vi "Teleop.vi"(10 "Match Info":T1={"Autonomous Elapsed Seconds"=0.0, "TeleOp Elapsed Seconds"=0.0, "Disabled Elapsed Seconds"=0.0, "Visited Autonomous"=FALSE, "Visited TeleOp"=FALSE, "Visited Disabled"=FALSE, "Autonomous Settings"={"Autonomous Style"=enum."Independent", "VI Refnum"=refnum}}, 11 "Call Context":T2) -> ()   [LabVIEW 2011]
doc: "This VI is called for each TeleOp packet received from the DS where the robot is not disabled. It is often used to read from the joysticks and update I/O or to update setpoints for timed control loops. It should complete and return within 20 milliseconds or it may miss DS packets."
uses:
  <vilib>/Rock Robotics/WPI/DriverStation/WPI_DriverStationDerivedRobotMode.ctl
  <vilib>/Rock Robotics/WPI/DriverStation/WPI_DriverStationMatch Info.ctl
  Robot Global Data.vi
panel:
  out "Right Speed":dbl
  out "Left Speed":dbl
  out "Hammer Speed":dbl
  out "Angle Speed":dbl
  in  "Test Shooter":bool
  out "Collector Speed":dbl
  out "Elevator Speed":dbl
  out "Shooter Speed":dbl
  # "Motot Inputs"
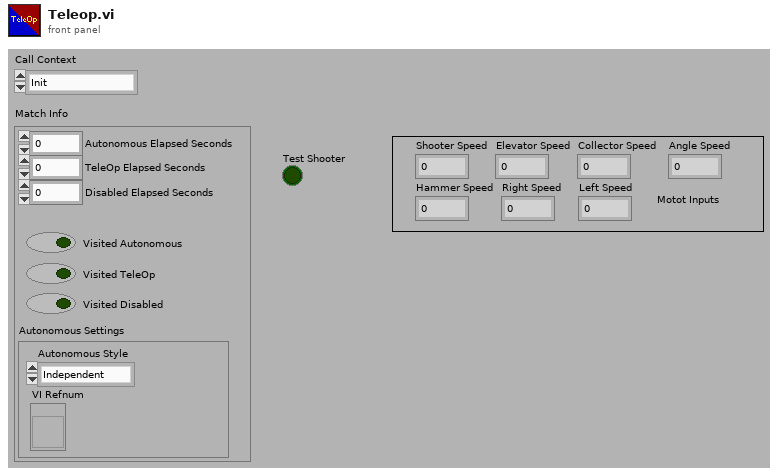
[diagram p1: front panel]
types:
  T1 = typedef "WPI_DriverStationMatch Info.ctl" = cluster{"Autonomous Elapsed Seconds":dbl, "TeleOp Elapsed Seconds":dbl, "Disabled Elapsed Seconds":dbl, "Visited Autonomous":bool, "Visited TeleOp":bool, "Visited Disabled":bool, "Autonomous Settings":cluster{"Autonomous Style":enum16{"Iterative", "Independent"}, "VI Refnum":refnum<vi>}}
  T2 = typedef "WPI_DriverStationDerivedRobotMode.ctl" = enum16{"Init", "Execute", "Stop"}
  T3 = typedef "WPI_JoystickDevRef.ctl" = cluster{"Device":T4}
  T4 = typedef "WPI_JoystickDeviceEnum.ctl" = enum16{"USB 1", "USB 2", "USB 3", "USB 4", "Kinect 1", "Kinect 2"}
  T5 = typedef "WPI_JoystickButtonState.ctl" = cluster{"Button 1":bool, "Button 2":bool, "Button 3":bool, "Button 4":bool, "Button 5":bool, "Button 6":bool, "Button 7":bool, "Button 8":bool, "Button 9":bool, "Button 10":bool, "Button 11":bool, "Button 12":bool}
  T6 = cluster{"axis 1 (x)":dbl, "axis 2 (y)":dbl, "axis 3 (throttle)":dbl, "axis 4":dbl, "axis 5":dbl, "axis 6":dbl}
  T7 = typedef "WPI_MotorControlDeviceRef.ctl" = cluster{"DeviceStatus":errorcluster, "Type":enum16{"PWM", "CAN"}, "PWM":cluster{"Digital Module":T8, "PWM Channel":T9, "DeadBand":T10}, "CAN":cluster{"Device Number":u8, "Control Mode":T11, "Semaphore":T12, "Max Vout":dbl}, "Invert":bool, "TransformRef":T13, "InvTransformRef":T13}
  T8 = typedef "FPGA_TypedefDigitalModule.ctl" = enum16{"Digital Module 1", "Digital Module 2"}
  T9 = typedef "FPGA_DIOPWMChannel.ctl" = enum8{"PWM 1", "PWM 2", "PWM 3", "PWM 4", "PWM 5", "PWM 6", "PWM 7", "PWM 8", "PWM 9", "PWM 10", "Invalid"}
  T10 = typedef "WPI_PWMDeadband.ctl" = cluster{"Name":string, "maxPositivePwm":i32, "minPositivePwm":i32, "centerPwm":i32, "maxNegativePwm":i32, "minNegativePwm":i32, "angularRange":u16}
  T11 = typedef "WPI_CANJaguar_ControlMode.ctl" = enum8{"Percent VBus", "Current", "Speed", "Position", "Voltage"}
  T12 = typedef "Semaphore RefNum" = refnum<k1>
  T13 = typedef "WPI_PWMTransform_ConPane.ctl" = refnum<vi>
  T14 = typedef "WPI_RobotDriveDevRef.ctl" = cluster{"DevStatus":errorcluster, "Motors[]":T7[], "Square Inputs":bool, "Max Output":dbl, "Isochronous":bool}
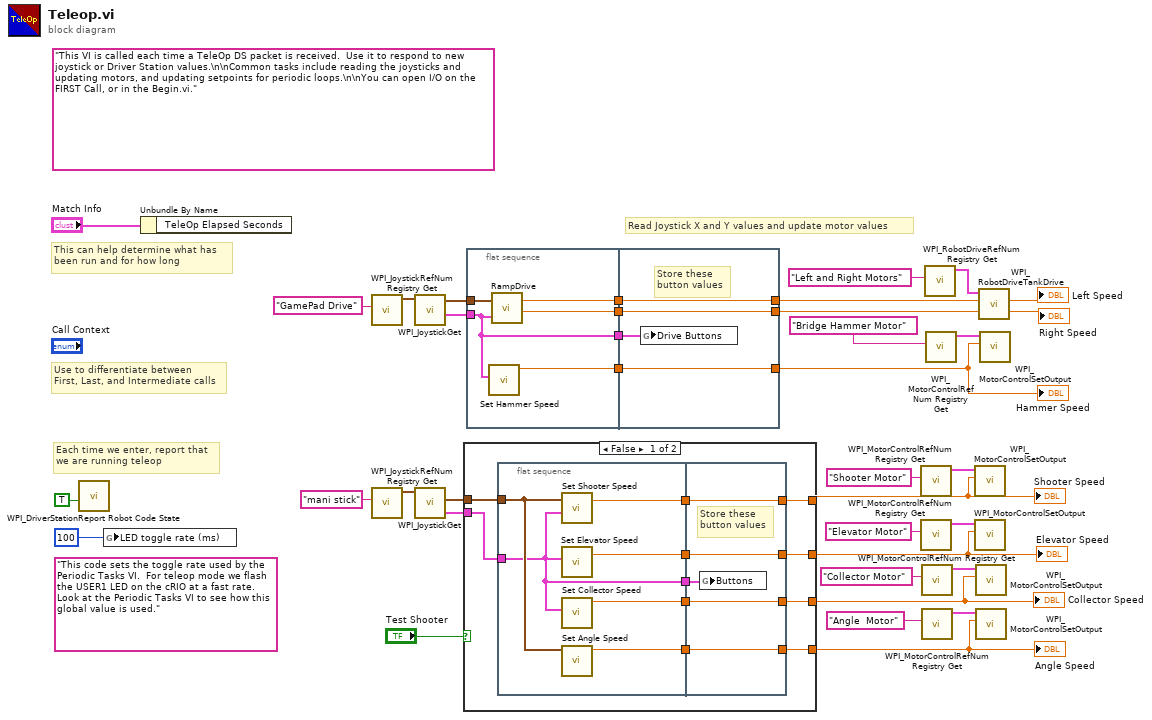
[diagram p0: block diagram]
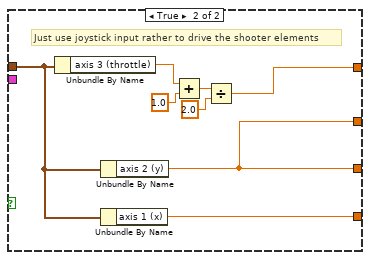
[diagram p2: hidden frame]
diagram:
  (unwired) "This code sets the toggle rate used by the Periodic Tasks VI.  For teleop mode we flash the USER1 LED on the cRIO at a fast rate.  Look at the Periodic Tasks VI to see how this global value is used."
  (unwired) "This VI is called each time a TeleOp DS packet is received.  Use it to respond to new joystick or Driver Station values.\n\nCommon tasks include reading the joysticks and updating motors, and updating setpoints for periodic loops.\n\nYou can open I/O on the FIRST Call, or in the Begin.vi."
  # "Each time we enter, report that\nwe are running teleop"
  # "Use to differentiate between\nFirst, Last, and Intermediate calls"
  # "This can help determine what has\nbeen run and for how long"
  # "Read Joystick X and Y values and update motor values"
  n1 = call <vilib>:"WPI_DriverStationReport Robot Code State.vi"("TeleOp"=TRUE ("Autonomous")) -> ()  [unwired: 10 in, 1 out]
  n2 = global write "Robot Global Data.vi" "LED toggle rate (ms)"(u32 100 ("LED ms toggle rate")) -> ()
  n3 = Unbundle By Name("Match Info") -> ()  [unwired: 1 out]
  n4 = call <vilib>:"WPI_JoystickRefNum Registry Get.vi"("refnum name"="GamePad Drive") -> ("JoystickDevRef"=w32:T3)  [unwired: 1 in, 9 out]
  n5 = call <vilib>:"WPI_JoystickRefNum Registry Get.vi"("refnum name"="mani stick") -> ("JoystickDevRef"=w24:T3)  [unwired: 9 in, 1 out]
  n6 = call <vilib>:"WPI_JoystickGet.vi"("JoystickDevRef"=w32) -> ("Buttons"=w19:T5, "Axes"=w28:T6)  [unwired: 1 in, 4 out]
  n7 = call <vilib>:"WPI_JoystickGet.vi"("JoystickDevRef"=w24) -> ("Buttons"=w22:T5, "Axes"=w23:T6)  [unwired: 4 in, 1 out]
  n8 = case shown="False" "Test Shooter" {
    tunnel: w23 -> [w42 w59]
    tunnel: [w46 w61] -> w3
    tunnel: [w45 w60] -> w4
    tunnel: w22 -> [w44 _]
    tunnel: [w43 w60] -> w5
    tunnel: [w41 w58] -> w6
    frame False {
      n9 = flat-sequence {
        tunnel: w44 -> [w47]
        tunnel: w42 -> [w49]
        tunnel: [w52] -> w40
        tunnel: [w51] -> w39
        tunnel: [w50] -> w38
        tunnel: [w48] -> w37
        tunnel: [w47] -> w36
        tunnel: [w54] -> w41
        tunnel: [w55] -> w43
        tunnel: [w56] -> w45
        tunnel: [w57] -> w46
        tunnel: w40 -> [w57]
        tunnel: w39 -> [w56]
        tunnel: w38 -> [w55]
        tunnel: w37 -> [w54]
        tunnel: w36 -> [w53]
        frame #0 {
          n10 = call "Set Shooter Speed.vi"("Buttons"=w47, "Axes"=w49) -> ("Shooter Speed"=w52:dbl)  [unwired: 9 in]
          n11 = call "Set Elevator Speed.vi"("Buttons"=w47) -> ("Elevator Speed"=w51:dbl)  [unwired: 10 in]
          n12 = call "Set Collector Speed.vi"("Buttons"=w47) -> ("Collector Speed"=w50:dbl)  [unwired: 10 in]
          n13 = call "Set Angle Speed.vi"("Axes"=w49) -> ("Angle Speed"=w48:dbl)  [unwired: 10 in]
        }
        frame #1 {
          # "Store these\nbutton values"
          n14 = global write "Robot Global Data.vi" "Buttons"(w53) -> ()
        }
      }
    }
    frame True {
      # "Just use joystick input rather to drive the shooter elements"
      n15 = Unbundle By Name(w59) -> ("axis 3 (throttle)"=w62:dbl)
      n16 = Unbundle By Name(w59) -> ("axis 2 (y)"=w60:dbl)
      n17 = Unbundle By Name(w59) -> ("axis 1 (x)"=w58:dbl)
      n18 = Add(x=w62, y=1.0) -> (x+y=w65:dbl)
      n19 = Divide(x=w65, y=2.0) -> (x/y=w61:dbl)
    }
  }
  "Shooter Speed" <- w3
  "Elevator Speed" <- w4
  "Collector Speed" <- w5
  "Angle Speed" <- w6
  n20 = flat-sequence {
    tunnel: w28 -> [w67]
    tunnel: w19 -> [w66]
    tunnel: [w69] -> w17
    tunnel: [w68] -> w16
    tunnel: [w70] -> w15
    tunnel: [w66] -> w14
    tunnel: [w71] -> w18
    tunnel: [w73] -> w26
    tunnel: [w74] -> w27
    tunnel: w17 -> [w74]
    tunnel: w16 -> [w73]
    tunnel: w15 -> [w71]
    tunnel: w14 -> [w72]
    frame #0 {
      n21 = call "Set Hammer Speed.vi"("Buttons"=w66) -> ("Hammer Speed"=w70:dbl)  [unwired: 10 in]
      n22 = call "RampDrive.vi"("Buttons"=w66, "Axes"=w67) -> ("Right Speed"=w68:dbl, "Left Speed"=w69:dbl)
    }
    frame #1 {
      # "Store these\nbutton values"
      n23 = global write "Robot Global Data.vi" "Drive Buttons"(w72) -> ()
    }
  }
  n24 = call <vilib>:"WPI_MotorControlRefNum Registry Get.vi"("refnum name"="Shooter Motor") -> ("MotorControlDevRef"=w12:T7)  [unwired: 9 in, 1 out]
  n25 = call <vilib>:"WPI_MotorControlRefNum Registry Get.vi"("refnum name"="Elevator Motor") -> ("MotorControlDevRef"=w10:T7)  [unwired: 9 in, 1 out]
  n26 = call <vilib>:"WPI_MotorControlRefNum Registry Get.vi"("refnum name"="Collector Motor") -> ("MotorControlDevRef"=w8:T7)  [unwired: 9 in, 1 out]
  n27 = call <vilib>:"WPI_MotorControlRefNum Registry Get.vi"("refnum name"="Angle  Motor") -> ("MotorControlDevRef"=w7:T7)  [unwired: 9 in, 1 out]
  n28 = call <vilib>:"WPI_RobotDriveRefNum Registry Get.vi"("refnum name"="Left and Right Motors") -> ("RobotDriveDevRef"=w29:T14)  [unwired: 1 in, 9 out]
  n29 = call <vilib>:"WPI_MotorControlRefNum Registry Get.vi"("refnum name"="Bridge Hammer Motor") -> ("MotorControlDevRef"=w20:T7)  [unwired: 9 in, 1 out]
  n30 = call <vilib>:"WPI_MotorControlSetOutput.vi"("Output"=w3, "MotorControlDevRef"=w12) -> ()  [unwired: 8 in, 2 out]
  n31 = call <vilib>:"WPI_MotorControlSetOutput.vi"("Output"=w4, "MotorControlDevRef"=w10) -> ()  [unwired: 8 in, 2 out]
  n32 = call <vilib>:"WPI_MotorControlSetOutput.vi"("Output"=w5, "MotorControlDevRef"=w8) -> ()  [unwired: 8 in, 2 out]
  n33 = call <vilib>:"WPI_MotorControlSetOutput.vi"("Output"=w6, "MotorControlDevRef"=w7) -> ()  [unwired: 8 in, 2 out]
  n34 = call <vilib>:"WPI_RobotDriveTankDrive.vi"("Right axis value"=w26, "Left axis value"=w27, "RobotDriveDevRef"=w29) -> ()  [unwired: 7 in, 2 out]
  n35 = call <vilib>:"WPI_MotorControlSetOutput.vi"("Output"=w18, "MotorControlDevRef"=w20) -> ()  [unwired: 8 in, 2 out]
  "Hammer Speed" <- w18
  "Left Speed" <- w27
  "Right Speed" <- w26
